vi "ParseJSON.vi"(8 "error in (no error)":errorcluster, 11 "JSON String":string) -> (0 "error out":errorcluster, 3 "JSONCluster":T1)   [LabVIEW 2015]
uses:
  Typedef/JSONCluster.ctl
  <vilib>/LVH/i3 JSON/JSON Parsing/Get Object Parameter Files/Get Object Parameter - Object.vi
  <vilib>/LVH/i3 JSON/JSON Parsing/Get Array Value at Index Files/Get Array Value at Index - Object.vi
  <vilib>/LVH/i3 JSON/i3-json.lvlib
panel:
  in  "Tree":string(tree)
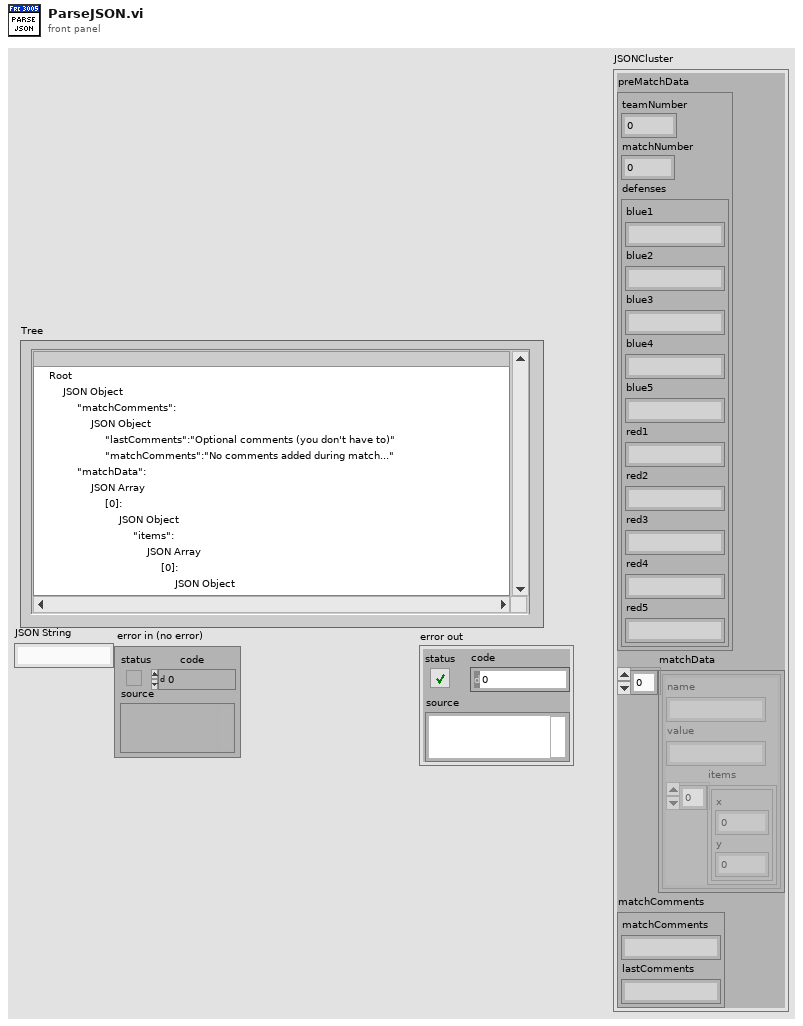
[diagram p1: front panel]
types:
  T1 = typedef "JSONCluster.ctl" = cluster{"preMatchData":cluster{"teamNumber":i32, "matchNumber":i32, "defenses":cluster{"blue1":string, "blue2":string, "blue3":string, "blue4":string, "blue5":string, "red1":string, "red2":string, "red3":string, "red4":string, "red5":string}}, "matchData":cluster{"name":string, "value":string, "items":cluster{"x":i32, "y":i32}[]}[], "matchComments":cluster{"matchComments":string, "lastComments":string}}
  T2 = cluster{"name":string, "value":string, "items":cluster{"x":i32, "y":i32}[]}
  T3 = cluster{"[0]":string, "[1]":string, "[2]":string, "[3]":string, "[4]":string, "[5]":string, "[6]":string, "[7]":string, "[8]":string, "[9]":string}
  T4 = cluster{i32, i32, cluster{"[0]":string, "[1]":string, "[2]":string, "[3]":string, "[4]":string, "[5]":string, "[6]":string, "[7]":string, "[8]":string, "[9]":string}}
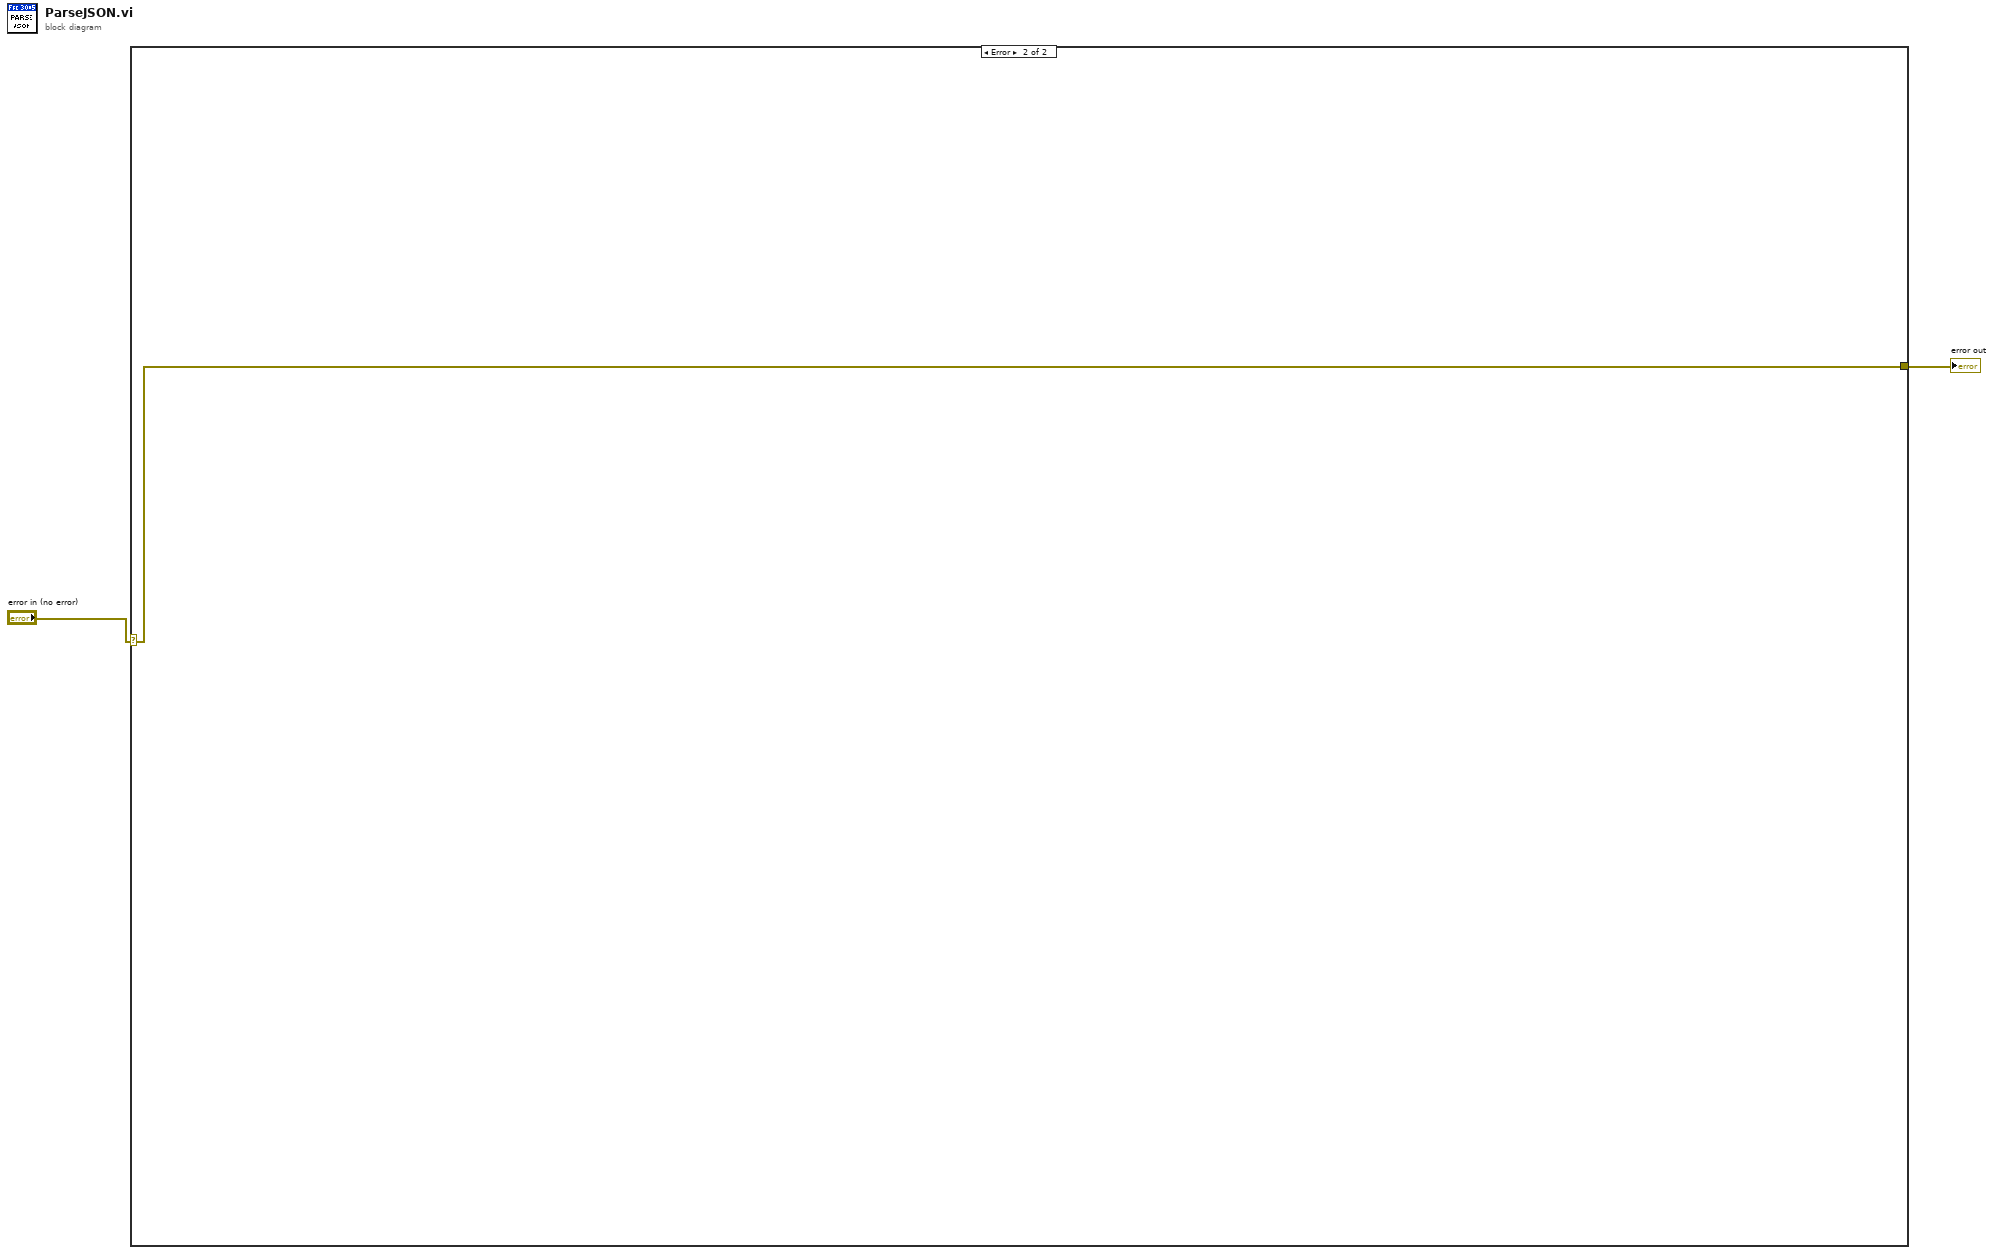
[diagram p0: block diagram]
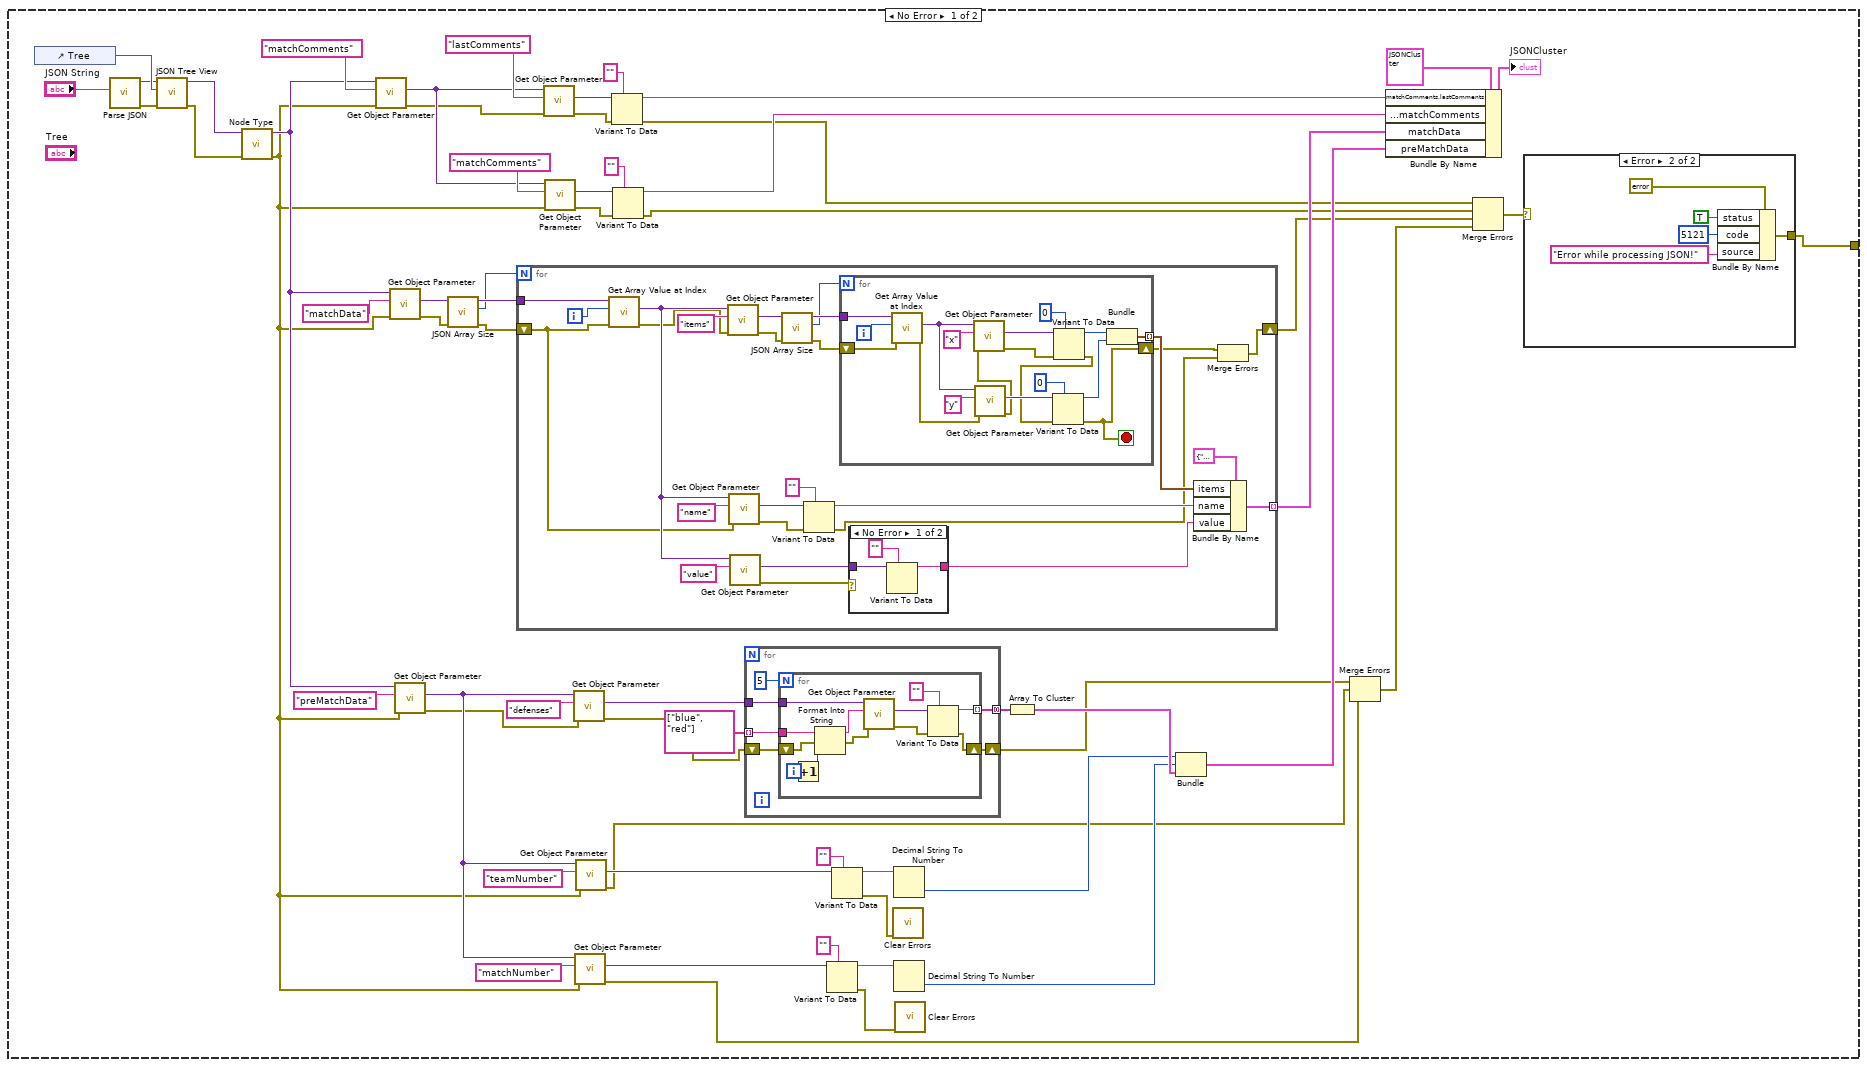
[diagram p2: hidden frame]
diagram:
  n1 = case shown="Error" "error in (no error)" {
    selector: "error in (no error)" -> [_ w134]
    tunnel: [w3 w134] -> w2
    frame No Error {
      n2 = control-ref of="Tree"() -> (w63:refnum<vi>)
      n3 = call <vilib>:"Parse JSON.vi"("JSON String"="JSON String") -> ("error out"=w21:errorcluster, "JSON Tree"=w62:variant)  [unwired: 7 in, 2 out]
      n4 = call <vilib>:"JSON Tree View.vi"("error in (no error)"=w21, "JSON Tree Expanded Reference"=w63, "JSON Tree"=w62) -> ("error out"=w20:errorcluster, "JSON Tree Passthrough"=w61:variant)  [unwired: 7 in]
      n5 = call <vilib>:"Node Type.vi"("error in (no error)"=w20, "JSON Tree In"=w61) -> ("error out"=w10:errorcluster, "JSON Tree Passthrough"=w42:variant)  [unwired: 5 in, 3 out]
      n6 = call-poly <vilib>:"Get Object Parameter.vi"("error in (no error)"=w10, "Parameter Name"="matchComments", "JSON Tree In (JSON Object)"=w42) -> ("error out"=w19:errorcluster, "JSON Object"=w50:variant)  [unwired: 5 in, 2 out]
      n7 = call-poly <vilib>:"Get Object Parameter.vi"("error in (no error)"=w10, "Parameter Name"="matchData", "JSON Tree In (JSON Object)"=w42) -> ("error out"=w16:errorcluster, "JSON Object"=w47:variant)  [unwired: 5 in, 2 out]
      n8 = call-poly <vilib>:"Get Object Parameter.vi"("error in (no error)"=w10, "Parameter Name"="preMatchData", "JSON Tree In (JSON Object)"=w42) -> ("error out"=w11:errorcluster, "JSON Object"=w38:variant)  [unwired: 5 in, 2 out]
      n9 = call <vilib>:"JSON Array Size.vi"("error in (no error)"=w16, "JSON Tree In (JSON Array)"=w47) -> ("error out"=w15:errorcluster, "Array Size"=w45:i32, "JSON Tree Passthrough (JSON Array)"=w46:variant)  [unwired: 7 in]
      n10 = for {
        N: w45 -> [_]
        tunnel: w46 -> [w112]
        tunnel: [w97] -> w44 mode=indexing
        shift-right: [w91] -> w12
        shift-left: w15 -> [w89]
        i -> [w111]
        n11 = call-poly <vilib>:"Get Array Value at Index.vi"("error in (no error)"=w89, "Index"=w111, "JSON Tree In (JSON Array)"=w112) -> ("error out"=w94:errorcluster, "JSON Object"=w107:variant)  [unwired: 5 in, 2 out]
        n12 = call-poly <vilib>:"Get Object Parameter.vi"("error in (no error)"=w94, "Parameter Name"="items", "JSON Tree In (JSON Object)"=w107) -> ("error out"=w93:errorcluster, "JSON Object"=w104:variant)  [unwired: 5 in, 2 out]
        n13 = call-poly <vilib>:"Get Object Parameter.vi"("error in (no error)"=w89, "Parameter Name"="name", "JSON Tree In (JSON Object)"=w107) -> ("error out"=w88:errorcluster, "JSON Object"=w105:variant)  [unwired: 5 in, 2 out]
        n14 = call-poly <vilib>:"Get Object Parameter.vi"("Parameter Name"="value", "JSON Tree In (JSON Object)"=w107) -> ("error out"=w101:errorcluster, "JSON Object"=w102:variant)  [unwired: 6 in, 2 out]
        n15 = call <vilib>:"JSON Array Size.vi"("error in (no error)"=w93, "JSON Tree In (JSON Array)"=w104) -> ("error out"=w92:errorcluster, "Array Size"=w96:i32, "JSON Tree Passthrough (JSON Array)"=w103:variant)  [unwired: 7 in]
        n16 = Variant To Data(error in=w88, type="", Variant=w105) -> (data=w98:string, error out=w87:errorcluster)
        n17 = for {
          N: w96 -> [_]
          tunnel: w103 -> [w132]
          tunnel: [w122] -> w99 mode=indexing
          shift-right: [w116] -> w90
          shift-left: w92 -> [w121]
          i -> [w133]
          stop <- w116 stop-if-true
          n18 = call-poly <vilib>:"Get Array Value at Index.vi"("error in (no error)"=w121, "Index"=w133, "JSON Tree In (JSON Array)"=w132) -> ("error out"=w120:errorcluster, "JSON Object"=w129:variant)  [unwired: 5 in, 2 out]
          n19 = call-poly <vilib>:"Get Object Parameter.vi"("error in (no error)"=w120, "Parameter Name"="y", "JSON Tree In (JSON Object)"=w129) -> ("error out"=w119:errorcluster, "JSON Object"=w127:variant)  [unwired: 5 in, 2 out]
          n20 = call-poly <vilib>:"Get Object Parameter.vi"("error in (no error)"=w119, "Parameter Name"="x", "JSON Tree In (JSON Object)"=w129) -> ("error out"=w118:errorcluster, "JSON Object"=w128:variant)  [unwired: 5 in, 2 out]
          n21 = Variant To Data(error in=w118, type=0 ("x"), Variant=w128) -> (data=w124:i32, error out=w117:errorcluster)
          n22 = Variant To Data(error in=w117, type=0 ("x"), Variant=w127) -> (data=w123:i32, error out=w116:errorcluster)
          n23 = Bundle("x"=w124, "x"=w123) -> (w122:cluster{"x":i32, "x":i32})  [unwired: 1 in]
        }
        n24 = case shown="No Error" w101 {
          tunnel: w102 -> [w114 _]
          tunnel: [w113 _] -> w95
          frame No Error {
            n25 = Variant To Data(type="", Variant=w114) -> (data=w113:string)  [unwired: 1 in, 1 out]
          }
          frame Error {
          }
        }
        n26 = Bundle By Name(cluster=T2 {"name"="", "value"="", "items"=[]}, "items"=w99, "name"=w98, "value"=w95) -> (w97:T2)
        n27 = Merge Errors(w90, w87) -> (w91:errorcluster)
      }
      n28 = call-poly <vilib>:"Get Object Parameter.vi"("error in (no error)"=w19, "Parameter Name"="lastComments", "JSON Tree In (JSON Object)"=w50) -> ("error out"=w18:errorcluster, "JSON Object"=w58:variant)  [unwired: 5 in, 2 out]
      n29 = call-poly <vilib>:"Get Object Parameter.vi"("error in (no error)"=w10, "Parameter Name"="matchComments", "JSON Tree In (JSON Object)"=w50) -> ("error out"=w17:errorcluster, "JSON Object"=w52:variant)  [unwired: 5 in, 2 out]
      n30 = call-poly <vilib>:"Get Object Parameter.vi"("error in (no error)"=w11, "Parameter Name"="defenses", "JSON Tree In (JSON Object)"=w38) -> ("error out"=w9:errorcluster, "JSON Object"=w37:variant)  [unwired: 5 in, 2 out]
      n31 = call-poly <vilib>:"Get Object Parameter.vi"("error in (no error)"=w10, "Parameter Name"="matchNumber", "JSON Tree In (JSON Object)"=w38) -> ("error out"=w6:errorcluster, "JSON Object"=w33:variant)  [unwired: 5 in, 2 out]
      n32 = call-poly <vilib>:"Get Object Parameter.vi"("error in (no error)"=w10, "Parameter Name"="teamNumber", "JSON Tree In (JSON Object)"=w38) -> ("error out"=w7:errorcluster, "JSON Object"=w34:variant)  [unwired: 5 in, 2 out]
      n33 = Variant To Data(error in=w18, type="", Variant=w58) -> (data=w55:string, error out=w14:errorcluster)
      n34 = Variant To Data(error in=w17, type="", Variant=w52) -> (data=w49:string, error out=w13:errorcluster)
      n35 = for {
        tunnel: w37 -> [w74]
        tunnel: string[] ["blue", "red"] -> [w72] mode=indexing
        tunnel: [w71] -> w35 mode=concatenating
        shift-right: [w70] -> w8
        shift-left: w9 -> [w69]
        n36 = for {
          N: 5 -> [_]
          tunnel: w74 -> [w83]
          tunnel: w72 -> [w85]
          tunnel: [w80] -> w71 mode=indexing
          shift-right: [w77] -> w70
          shift-left: w69 -> [w76]
          i -> [w86]
          n37 = Increment(x=w86) -> (x+1=w79:i32)
          n38 = Format Into String(initial string=w85, error in=w76, w79) -> (resulting string=w84:string, error out=w75:errorcluster)  [unwired: 1 in]
          n39 = call-poly <vilib>:"Get Object Parameter.vi"("error in (no error)"=w75, "Parameter Name"=w84, "JSON Tree In (JSON Object)"=w83) -> ("error out"=w78:errorcluster, "JSON Object"=w81:variant)  [unwired: 5 in, 2 out]
          n40 = Variant To Data(error in=w78, type="", Variant=w81) -> (data=w80:string, error out=w77:errorcluster)
        }
      }
      n41 = Variant To Data(type="", Variant=w33) -> (data=w31:string, error out=w23:errorcluster)  [unwired: 1 in]
      n42 = Variant To Data(type="", Variant=w34) -> (data=w32:string, error out=w24:errorcluster)  [unwired: 1 in]
      n43 = call <vilib>:"Clear Errors.vi"("error in (no error)"=w24) -> ()  [unwired: 5 in, 2 out]
      n44 = Decimal String To Number(string=w32) -> (number=w25:i32)  [unwired: 2 in, 1 out]
      n45 = Decimal String To Number(string=w31) -> (number=w26:i32)  [unwired: 2 in, 1 out]
      n46 = call <vilib>:"Clear Errors.vi"("error in (no error)"=w23) -> ()  [unwired: 5 in, 2 out]
      n47 = Array To Cluster(array=w35) -> (cluster=w30:T3)
      n48 = Bundle(w25, w26, w30) -> (w29:T4)  [unwired: 1 in]
      n49 = Merge Errors(w8, w7, w6) -> (w5:errorcluster)
      n50 = Bundle By Name(cluster=T1 {"preMatchData"={"teamNumber"=0, "matchNumber"=0, "defenses"={"blue1"="", "blue2"="", "blue3"="", "blue4"="", "blue5"="", "red1"="", "red2"="", "red3"="", "red4"="", "red5"=""}}, "matchData"=[], "matchComments"={"matchComments"="", "lastComments"=""}} ("JSONCluster"), "matchComments.lastComments"=w55, "matchComments.matchComments"=w49, "matchData"=w44, "preMatchData"=w29) -> (→"JSONCluster":T1)
      n51 = Merge Errors(w14, w13, w12, w5) -> (w4:errorcluster)
      n52 = case shown="Error" w4 {
        tunnel: [_ w67] -> w3
        frame No Error {
        }
        frame Error {
          n53 = Bundle By Name(cluster=errorcluster {"status"=FALSE, "code"=0, "source"=""} ("error in (no error)"), "status"=TRUE, "code"=5121, "source"="Error while processing JSON!") -> (w67:errorcluster)
        }
      }
    }
    frame Error {
    }
  }
  "error out" <- w2
